vi "Lucky Draw.vi"() -> ()   [LabVIEW 2020]
panel:
  out "s? t:f":string
  out "Lucky Number":i32
  in  "Run":i32
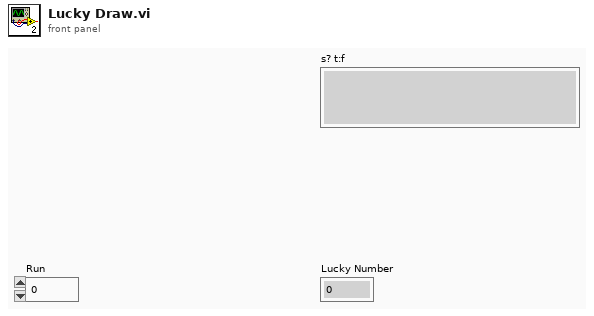
[diagram p1: front panel]
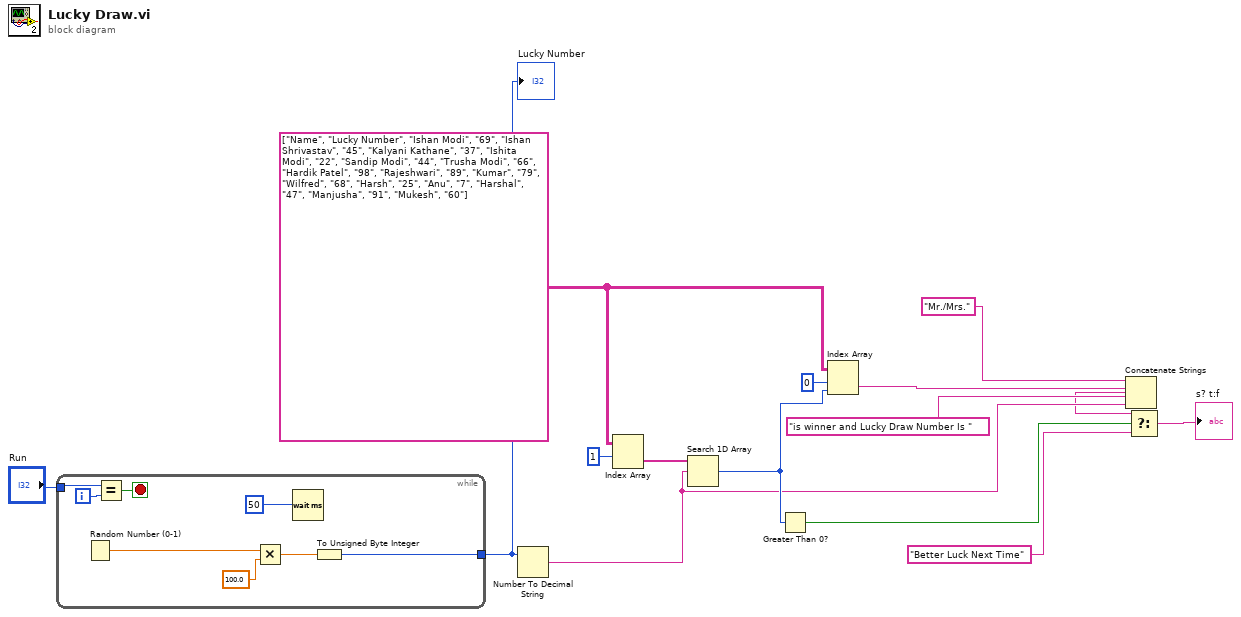
[diagram p0: block diagram]
diagram:
  w11 = string[][] [["Name", "Lucky Number"], ["Ishan Modi", "69"], ["Ishan Shrivastav", "45"], ["Kalyani Kathane", "37"], ["Ishita Modi", "22"], ["Sandip Modi", "44"], ["Trusha Modi", "66"], ["Hardik Patel", "98"], ["Rajeshwari", "89"], ["Kumar", "79"], ["Wilfred", "68"], ["Harsh", "25"], ["Anu", "7"], ["Harshal", "47"], ["Manjusha", "91"], ["Mukesh", "60"]]
  n1 = while {
    tunnel: "Run" -> [w20]
    tunnel: [w17] -> w12
    i -> [w19]
    stop <- w18 stop-if-true
    n2 = Random Number (0-1)() -> (number: 0 to 1=w23:dbl)
    n3 = Equal?(x=w20, y=w19) -> (x = y?=w18:bool)
    n4 = Multiply(x=w23, y=100.0) -> (x*y=w21:dbl)
    n5 = Wait (ms)(milliseconds to wait=50) -> ()  [unwired: 1 out]
    n6 = To Unsigned Byte Integer(number=w21) -> (unsigned 8bit integer=w17:u8)
  }
  "Lucky Number" <- w12
  n7 = Number To Decimal String(number=w12) -> (decimal integer string=w3:string)  [unwired: 1 in]
  n8 = Index Array "Index Array"(array=w11, index (row)=1) -> (element=w13:string[])  [unwired: 1 in]
  n9 = Search 1D Array(1D array=w13, element=w3) -> (index of element=w9:i32)  [unwired: 1 in]
  n10 = Greater Than 0?(x=w9) -> (x > 0?=w8:bool)
  n11 = Index Array "Index Array"(array=w11, index (row)=0, index (col)=w9) -> (element=w5:string)
  n12 = Concatenate Strings("Mr./Mrs.", w5, "is winner and Lucky Draw Number Is ", w3) -> (w2:string)
  n13 = Select(t=w2, s=w8, f="Better Luck Next Time") -> (s? t:f=→"s? t:f":string)
